vi "inv kin.vi"(10 "Kinematics Param":T1={"Length of arms \"a\" (cm)"=8.0, "Length of arms \"b\" (cm)"=16.0, "Length of  base \"r\" (cm)"=2.875, "Length of platform \"h\" (cm)"=1.5, "Phi (deg)"=[-150.0, -30.0, 90.0], "Upper limit of Theta"=0.0, "Lower limit of Theta"=0.0}, 11 "Point of TCF (X,Y,Z)":dbl[](array[numeric])=[1.0, 0.0, 17.2]) -> (1 "inRange":bool, 2 "Debug":dbl[](array[numeric]), 3 "Theta (deg)":dbl[](array[numeric])=[30.57465073099771, 23.96731469481936, 27.31346671314327])   [LabVIEW 2014]
uses:
  Kimematics Param.ctl
panel:
  # "Robot Diagram (single arm)"
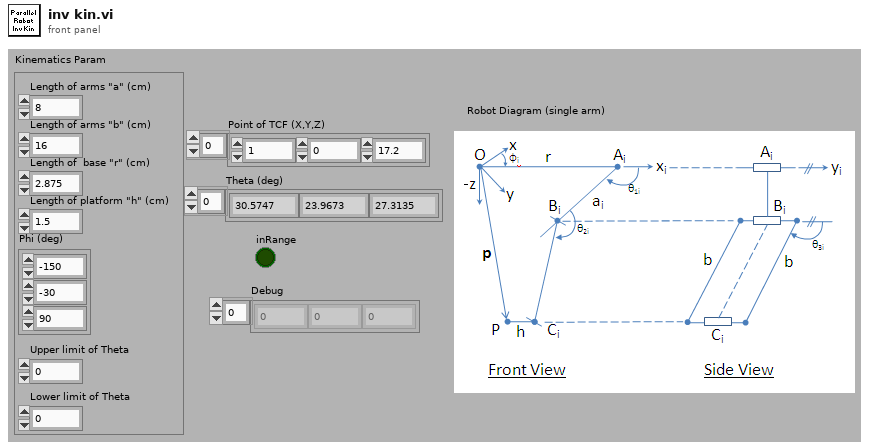
[diagram p1: front panel]
types:
  T1 = typedef "Kimematics Param.ctl" = cluster{"Length of arms \"a\" (cm)":dbl, "Length of arms \"b\" (cm)":dbl, "Length of  base \"r\" (cm)":dbl, "Length of platform \"h\" (cm)":dbl, "Phi (deg)":dbl[], "Upper limit of Theta":dbl, "Lower limit of Theta":dbl}
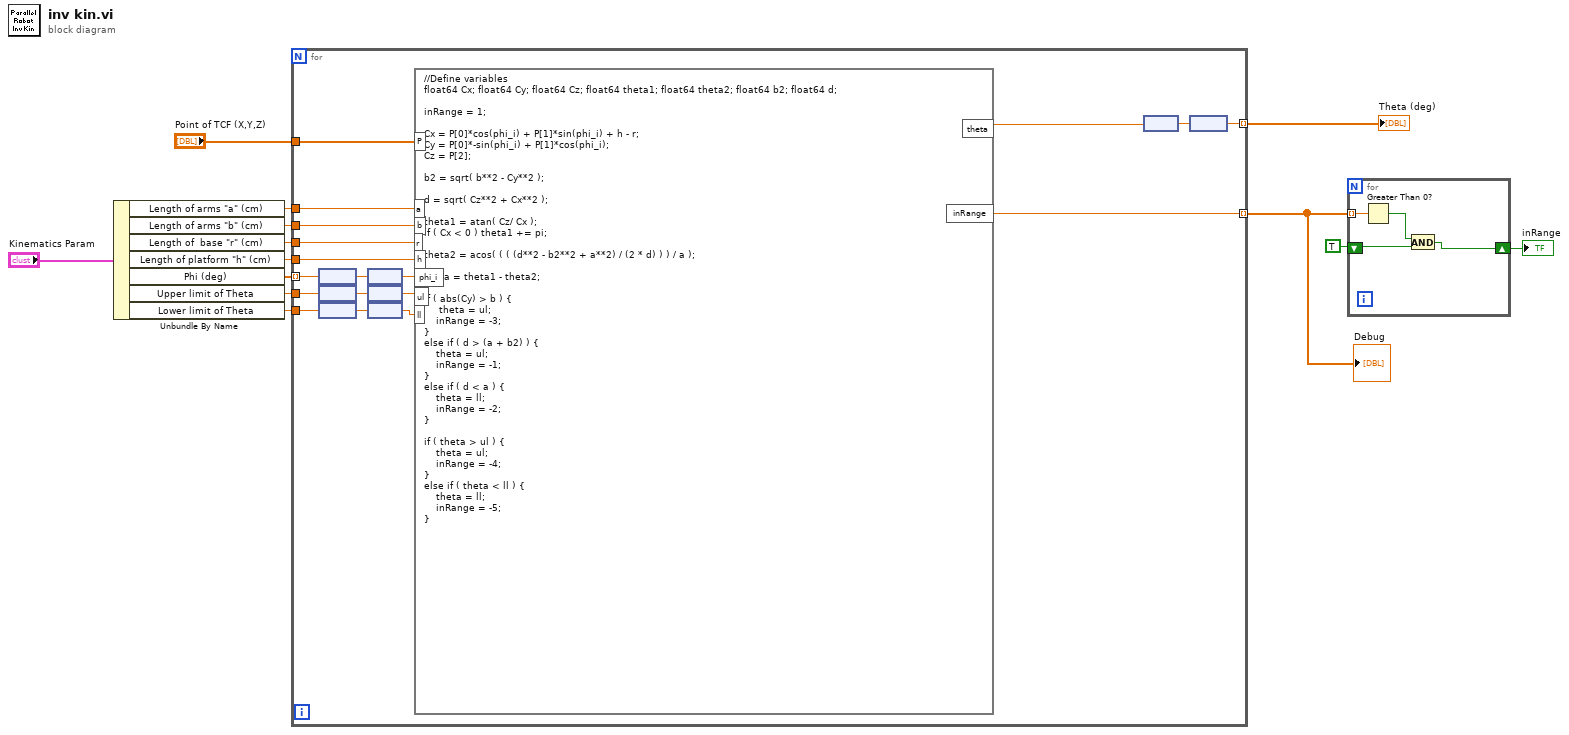
[diagram p0: block diagram]
diagram:
  n1 = Unbundle By Name("Kinematics Param") -> ("Length of arms \"a\" (cm)"=w8:dbl, "Length of arms \"b\" (cm)"=w11:dbl, "Length of  base \"r\" (cm)"=w10:dbl, "Length of platform \"h\" (cm)"=w9:dbl, "Phi (deg)"=w7:dbl[], "Upper limit of Theta"=w5:dbl, "Lower limit of Theta"=w4:dbl)
  n2 = for {
    tunnel: "Point of TCF (X,Y,Z)" -> [w31]
    tunnel: w11 -> [w28]
    tunnel: w10 -> [w29]
    tunnel: w9 -> [w30]
    tunnel: w7 -> [w24] mode=indexing
    tunnel: [w22] -> w13 mode=indexing
    tunnel: w8 -> [w27]
    tunnel: w5 -> [w15]
    tunnel: w4 -> [w14]
    tunnel: [w21] -> w3 mode=indexing
    n3 = node(w24) -> (w25:dbl[unit])
    n4 = node(w15) -> (w20:dbl[unit])
    n5 = node(w14) -> (w18:dbl[unit])
    n6 = node(w25) -> (w23:dbl)
    n7 = node(w20) -> (w19:dbl)
    n8 = node(w18) -> (w17:dbl)
    n9 = formula code="//Define variables\nfloat64 Cx; float64 Cy; float64 Cz; float64 theta1; float64 theta2; float64 b2; float64 d;\n\ninRange = 1;\n\nCx = P[0]*cos(phi_i) + P[1]*sin(phi_i) + h - r;\nCy = P[0]*-sin(phi_i) + P[1]*cos(phi_i);\nCz = P[2];\n\nb2 = sqrt( b**2 - Cy**2 );\n\nd = sqrt( Cz**2 + Cx**2 );\n\ntheta1 = atan( Cz/ Cx );\nif ( Cx < 0 ) theta1 += pi;\n\ntheta2 = acos( ( ( (d**2 - b2**2 + a**2) / (2 * d) ) ) / a );\n\ntheta = theta1 - theta2;\n\nif ( abs(Cy) > b ) {\n     theta = ul;\n    inRange = -3;\n}\nelse if ( d > (a + b2) ) {\n    theta = ul;\n    inRange = -1;\n}\nelse if ( d < a ) {\n    theta = ll;\n    inRange = -2;\n}\n\nif ( theta > ul ) {\n    theta = ul;\n    inRange = -4;\n}\nelse if ( theta < ll ) {\n    theta = ll;\n    inRange = -5;\n}"("P"=w31, "b"=w28, "r"=w29, "h"=w30, "phi_i"=w23, "a"=w27, "ul"=w19, "ll"=w17) -> ("theta"=w16:dbl, "inRange"=w21:dbl)
    n10 = node(w16) -> (w26:dbl[unit])
    n11 = node(w26) -> (w22:dbl)
  }
  "Theta (deg)" <- w13
  "Debug" <- w3
  n12 = for {
    tunnel: w3 -> [w35] mode=indexing
    shift-right: [w32] -> w1
    shift-left: TRUE -> [w33]
    n13 = Greater Than 0?(x=w35) -> (x > 0?=w34:bool)
    n14 = And(x=w34, y=w33) -> (x .and. y?=w32:bool)
  }
  "inRange" <- w1
